vi "Capacitance_VoltageRampTest.vi"(6 "Peak duration (s)":dbl, 9 "DCPower_Sequence_Parameters":T1[](array[typedef]) {"DeltaVoltage" format="%.6p"; "DeltaTime" format="%.6p"; "Voltage Stop" format="%.6p"; "Aperture_time" format="%.6p"; "Current_range" format="%.6p"; "Current" format="%.6p"; "Voltage_range" format="%.6p"; "Voltage Start" format="%.6p"}, 10 "Pins":T3[](array[typedef]), 11 "Semiconductor Module Context":T2) -> (0 "error out":errorcluster)   [LabVIEW 2023, in "Capacitance.lvlib"]
doc: "Calculates the Capacitance using the Voltage Ramp method.\nThe SMU generates a Voltage step and during the rising edge the Capacitance is calculated using the formula C=I*dt/dV"
uses:
  Capacitance.lvlib
  <vilib>/NI_TestStand_SemiconductorModule/NI_TestStand_Semiconductor_Module.lvlibp/PinMap/TagProvider/TSM_Pin.ctl
  <vilib>/NI_TestStand_SemiconductorModule/NI_TestStand_Semiconductor_Module.lvlibp/PinMap/General/SemiconductorModuleContext.ctl
  ResourceHandling/TypeDefs/RH_DCPower_SequenceParameters.ctl
  <vilib>/NI_TestStand_SemiconductorModule/NI_TestStand_Semiconductor_Module.lvlibp/PinMap/PinQueryContext/MultiplePinMultipleSessionQueryContext/MultiplePinMultipleSessionQueryContext.lvclass
  C:/Program Files/National Instruments/LabVIEW 2023/vi.lib/NI_TestStand_SemiconductorModule/NI_TestStand_Semiconductor_Module.lvlibp/PinMap/PinQueryContext/PinQueryContext.lvclass
  <vilib>/NI_TestStand_SemiconductorModule/NI_TestStand_Semiconductor_Module.lvlibp/PinMap/DC Power/PinsToNIDCPowerSessions.vi
  <vilib>/NI_TestStand_SemiconductorModule/NI_TestStand_Semiconductor_Module.lvlibp/PinMap/General/Publish/PublishDataDouble1D.vi
  <vilib>/NI_TestStand_SemiconductorModule/NI_TestStand_Semiconductor_Module.lvlibp
  ResourceHandling/ResourceHandling.lvlib
  C:/Program Files/National Instruments/LabVIEW 2023/vi.lib/NI_TestStand_SemiconductorModule/NI_TestStand_Semiconductor_Module.lvlibp/PinMap/PinQueryContext/MultipleSessionPinQueryContext.lvclass
  C:/Program Files/National Instruments/LabVIEW 2023/vi.lib/NI_TestStand_SemiconductorModule/NI_TestStand_Semiconductor_Module.lvlibp/PinMap/PinQueryContext/MultiplePinMultipleSessionQueryContext/MultiplePinMultipleSessionQueryContext.lvclass
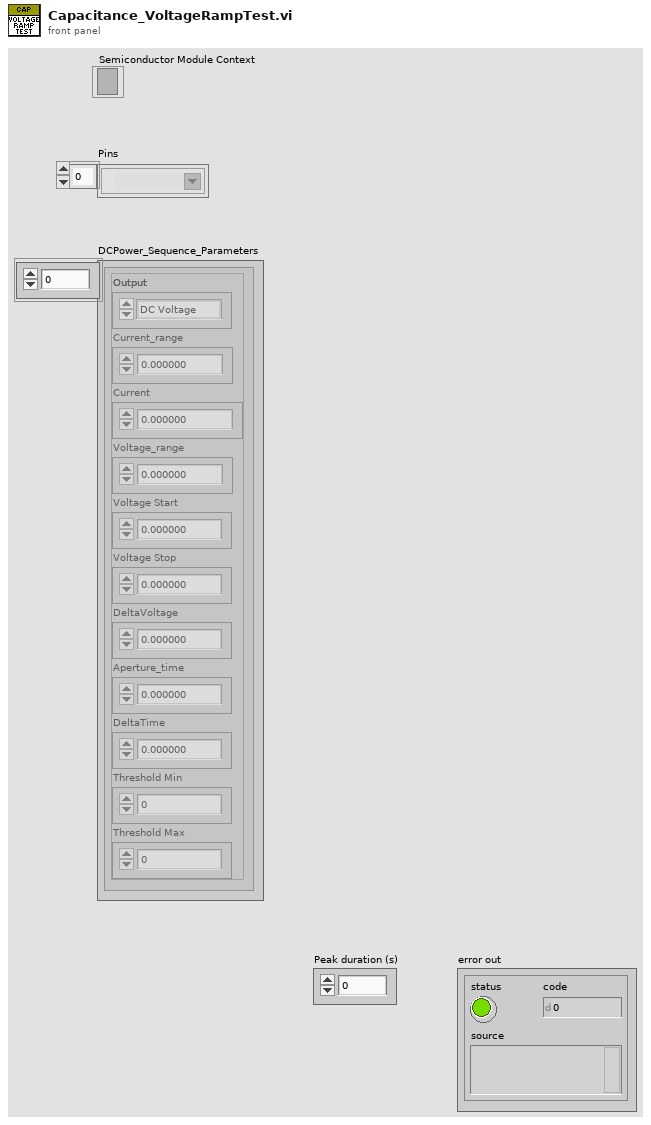
[diagram p1: front panel]
types:
  T1 = typedef "ResourceHandling.lvlib/RH_DCPower_SequenceParameters.ctl" = cluster{"Output":enum16{"DC Voltage", "DC Current"}, "Current_range":dbl, "Current":dbl, "Voltage_range":dbl, "Voltage Start":dbl, "Voltage Stop":dbl, "DeltaVoltage":dbl, "Aperture_time":dbl, "DeltaTime":dbl, "Threshold Min":dbl, "Threshold Max":dbl}
  T2 = typedef "NI_TestStand_Semiconductor_Module.lvlibp/SemiconductorModuleContext.ctl" = refnum<k7>
  T3 = typedef "NI_TestStand_Semiconductor_Module.lvlibp/TSM_Pin.ctl" = tag
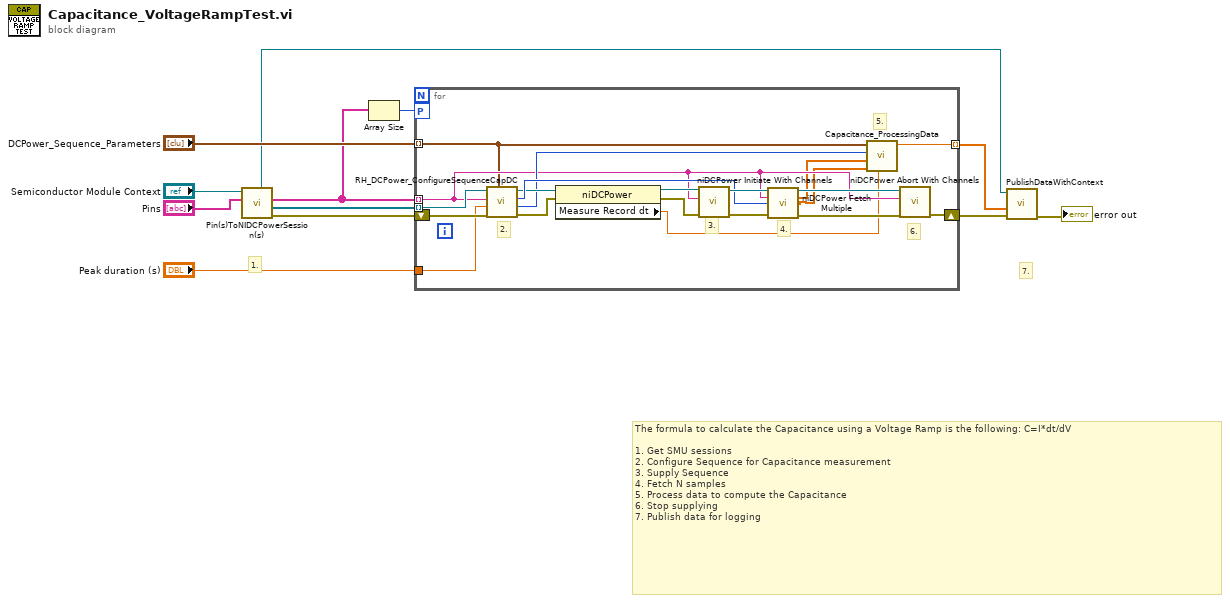
[diagram p0: block diagram]
diagram:
  # "7."
  # "The formula to calculate the Capacitance using a Voltage Ramp is the following: C=I*dt/dV\n\n1. Get SMU sessions\n2. Configure Sequence for Capacitance measurement\n3. Supply Sequence\n4. Fetch N samples\n5. Process data to compute the Capacitance\n6. Stop supplying\n7. Publish data for logging"
  # "1."
  n1 = call-poly <vilib>:"Pin(s)ToNIDCPowerSession(s).vi"("Pins"="Pins", "Semiconductor Module Context"="Semiconductor Module Context") -> ("error out"=w9:errorcluster, "Instrument Sessions"=w10:refnum<k15>[], "Channel Strings"=w1:string[], "Pin Query Context"=w4:refnum<class "MultiplePinMultipleSessionQueryContext.lvclass">)  [unwired: 5 in, 1 out]
  n2 = Array Size(array=w1) -> (size(s)=w2:i32)
  n3 = for {
    tunnel: w1 -> [w20] mode=indexing
    tunnel: w10 -> [w32] mode=indexing
    shift-right: [w14] -> w5
    shift-left: w9 -> [w31]
    tunnel: "DCPower_Sequence_Parameters" -> [w18] mode=indexing
    tunnel: "Peak duration (s)" -> [w30]
    tunnel: [w13] -> w3 mode=indexing
    workers-P: w2 -> [_]
    # "6."
    # "5."
    # "4."
    # "3."
    # "2."
    n4 = call "RH_DCPower_ConfigureSequenceCapDC.vi"("DCPower_SequenceParameters"=w18, "error in (no error)"=w31, "Peak duration (s)"=w30, "channel name"=w20, "DCPower Session In"=w32) -> ("error out"=w24:errorcluster, "RecordLength"=w22:i32, "num points"=w27:i32, "DCPower Session Out"=w26:refnum<k15>)  [unwired: 3 in]
    n5 = property class="niDCPower"(reference=w26, error in=w24) -> (reference out=w25:refnum<k15>, error out=w23:errorcluster, "Measure Record dt"=w15:dbl)
    n6 = call <instrlib>:"niDCPower Initiate With Channels.vi"("error in (no error)"=w23, "channel name"=w20, "instrument handle"=w25) -> ("error out"=w29:errorcluster, "instrument handle out"=w28:refnum<k15>)  [unwired: 7 in]
    n7 = call <instrlib>:"niDCPower Fetch Multiple.vi"("instrument handle"=w28, "channel name"=w20, "count (1)"=w27, "error in (no error)"=w29) -> ("instrument handle out"=w21:refnum<k15>, "voltage measurements"=w17:dbl[], "current measurements"=w16:dbl[], "error out"=w19:errorcluster)  [unwired: 6 in, 2 out]
    n8 = call "Capacitance_ProcessingData.vi"("Measure Record dt"=w15, "current measurements"=w16, "voltage measurements"=w17, "RecordLength"=w22, "DCPower_SequenceParameters"=w18) -> ("Capacitance"=w13:dbl)  [unwired: 6 in]
    n9 = call <instrlib>:"niDCPower Abort With Channels.vi"("error in (no error)"=w19, "channel name"=w20, "instrument handle"=w21) -> ("error out"=w14:errorcluster)  [unwired: 7 in, 1 out]
  }
  n10 = call-poly <vilib>:"PublishDataWithContext.vi"("error in (no error)"=w5, "Data In"=w3, "Pin Query Context"=w4) -> ("error out"=→"error out":errorcluster)  [unwired: 7 in, 1 out]
